vi "Check myRIO Status.vi"(8 "Error In":errorcluster) -> (0 "Error Out":errorcluster, 3 "myRIO Support Status":enum16{"Enabled", "Disabled"}(ring))   [LabVIEW 2013, in "LVH-LINX.lvlib"]
uses:
  <vilib>/LabVIEW Hacker/LINX/LVH-LINX.lvlib
  <vilib>/Utility/traverseref.llb/VI Scripting - Traverse.lvlib
  <vilib>/Utility/traverseref.llb/TRef TravTarget.ctl
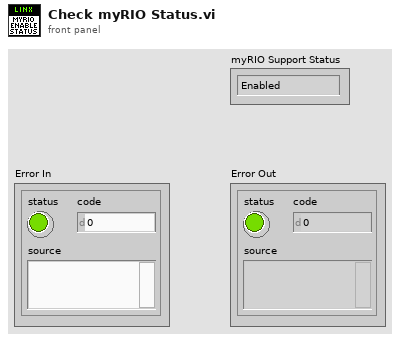
[diagram p1: front panel]
types:
  T1 = typedef "TRef TravTarget.ctl" = enum16{"FP", "BD", "Other"}
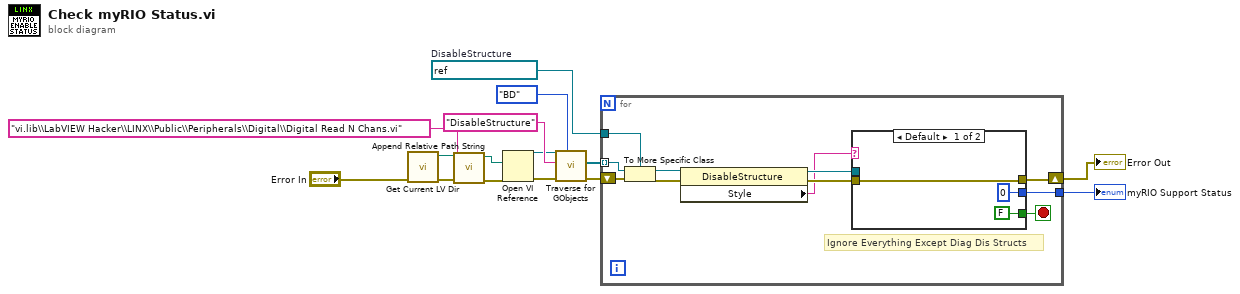
[diagram p0: block diagram]
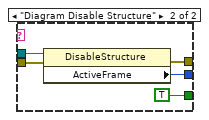
[diagram p2: hidden frame]
diagram:
  w11 = refnum<vi> refnum  # DisableStructure
  n1 = call <vilib>:"Get Current LV Dir.vi"("Error In"="Error In") -> ("Error Out"=w5:errorcluster, "This LV Directory"=w15:path)  [unwired: 9 in]
  n2 = call <vilib>:"Append Relative Path String.vi"("Error In"=w5, "Relative Path"="vi.lib\\LabVIEW Hacker\\LINX\\Public\\Peripherals\\Digital\\Digital Read N Chans.vi", "Base Path"=w15) -> ("Error Out"=w6:errorcluster, "Absolute Path"=w3:path)  [unwired: 7 in]
  n3 = Open VI Reference(vi path=w3, error in (no error)=w6) -> (vi reference=w8:refnum<vi>, error out=w13:errorcluster)  [unwired: 4 in]
  n4 = call <vilib>:"Traverse for GObjects.vi"("Traverse Target"=TRef_TravTarget."BD", "error in (no error)"=w13, "Class Name"="DisableStructure", "VI Refnum"=w8) -> ("error out"=w12:errorcluster, "References"=w7:refnum<vi>[])  [unwired: 4 in, 2 out]
  n5 = for {
    tunnel: w11 -> [w25]
    tunnel: w7 -> [w24] mode=indexing
    shift-right: [w23] -> w1
    shift-left: w12 -> [w26]
    tunnel: [w17] -> w2
    stop <- w16 stop-if-true
    # "Ignore Everything Except Diag Dis Structs"
    n6 = To More Specific Class(target class=w25, reference=w24, error in=w26) -> (specific class reference=w20:refnum<vi>, error out=w22:errorcluster)
    n7 = property class="DisableStructure"(reference=w20, error in=w22) -> (reference out=w19:refnum<vi>, error out=w21:errorcluster, "Style"=w18:string)
    n8 = case shown="Default" w18 {
      tunnel: [w29 w34] -> w23
      tunnel: w21 -> [w29 w33]
      tunnel: w19 -> [_ w32]
      tunnel: [i16 0 ("ActiveFrame") w31] -> w17
      tunnel: [FALSE TRUE] -> w16
      frame Default {
      }
      frame "Diagram Disable Structure" {
        n9 = property class="DisableStructure"(reference=w32, error in=w33) -> (error out=w34:errorcluster, "ActiveFrame"=w31:i16)  [unwired: 1 out]
      }
    }
  }
  "myRIO Support Status" <- w2
  "Error Out" <- w1
